vi "Loop Async.vi"(10 "ExecAnchor":refnum<class "ExecAnchor.lvclass">, 11 "Basic WebSocket Manager in":refnum<class "Basic WebSocket Manager.lvclass">) -> ()   [LabVIEW 2020, in "HTTP Server.lvlib" / "Basic WebSocket Manager.lvclass"]
uses:
  Basic WebSocket Manager.lvclass
  Basic WebSocket Manager.lvclass/Basic WebSocket Manager.ctl
  lv-exec-anchor/ExecAnchor/ExecAnchor.lvclass
  WebSocket Client/WebSocket Client.lvclass
  lv-promises/Promises/Promise/Promise.lvclass
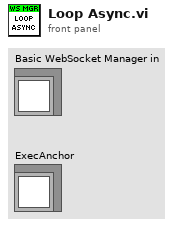
[diagram p1: front panel]
types:
  T1 = cluster{"Event Reg":refnum<event-registration>, "Event Reg":refnum<event-registration>}
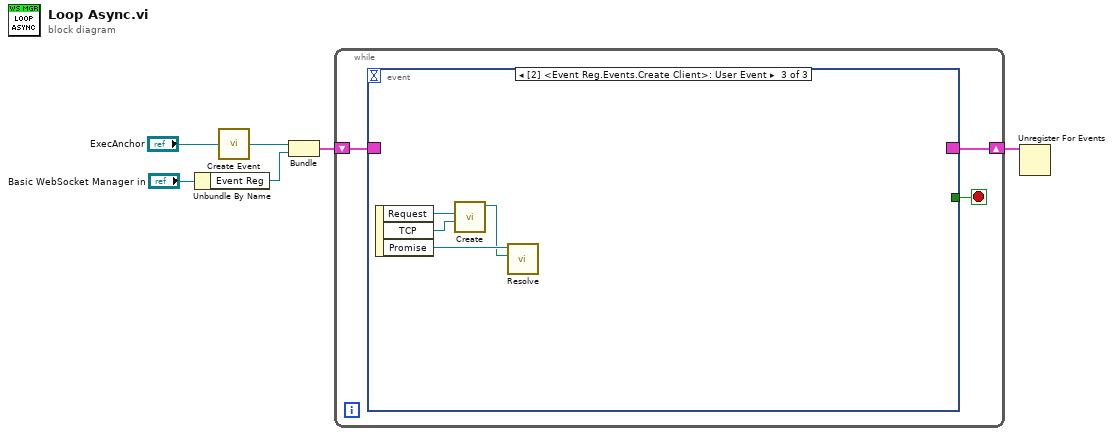
[diagram p0: block diagram]
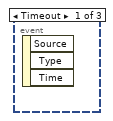
[diagram p2: hidden frame]
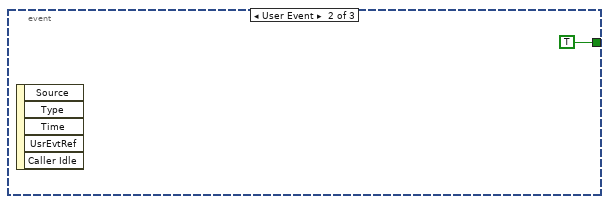
[diagram p3: hidden frame]
diagram:
  n1 = Unbundle By Name("Basic WebSocket Manager in") -> ("Event Reg"=w3:refnum<event-registration>)
  n2 = call "Create Event.vi"("ExecAnchor in"="ExecAnchor") -> ("Event Reg"=w4:refnum<event-registration>)  [unwired: 3 in, 1 out]
  n3 = Bundle("Event Reg"=w4, "Event Reg"=w3) -> (w2:T1)  [unwired: 1 in]
  n4 = while {
    shift-right: [w8] -> w1
    shift-left: w2 -> [w9]
    stop <- w7 stop-if-true
    n5 = event shown="[2] <Event Reg.Events.Create Client>: User Event" {
      selector: w9 -> [_ _ _]
      dyn-events: [_ _ _] -> w8
      timeout: _ -> [_ _ _]
      tunnel: [_ TRUE _] -> w7
      event Timeout {
        n6 = event-data() -> ()  [unwired: 1 in, 3 out]
      }
      event User Event {
        n7 = event-data() -> ()  [unwired: 1 in, 5 out]
      }
      event User Event {
        n8 = event-data() -> ("Request"=w14:refnum<class "Request.lvclass">, "TCP"=w13:refnum<k5>, "Promise"=w12:refnum<class "Promise.lvclass">)  [unwired: 1 in]
        n9 = call "Create.vi"("TCP"=w13, "Request"=w14) -> ("WebSocket Client out"=w11:refnum<class "WebSocket Client.lvclass">)  [unwired: 8 in, 1 out]
        n10 = call "Resolve.vi"("Result (None)"=w11, "Promise in"=w12) -> ()  [unwired: 8 in, 2 out]
      }
    }
  }
  n11 = Unregister For Events(event registration refnum=w1) -> ()  [unwired: 1 in, 1 out]
